vi "programmaticbuild2.vi"() -> ()   [LabVIEW 2015]
doc: "This VI reads an unlimited number of parameters corresponding to project files to build. To build projects programmatically, enter the following text in the command line window to run this VI:\n\n<LabVIEW directory>\\labview.exe \"<this VI>\" -- \"<project file 1>.lvproj\" \"<project file 2>.lvproj\" ... \"<project file n>.lvproj\"\n\nRefer to the block diagram for more information about how this VI executes."
panel:
  out "Built Successfully?":bool
  out "Currently building project":string
  # "Select Help»Show Context Help and move the cursor over the VI icon to display help for this VI."
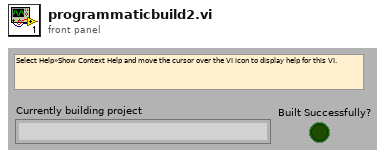
[diagram p1: front panel]
types:
  T1 = enum16{"open", "replace", "create", "open or create", "replace or create", "replace or create with confirmation"}
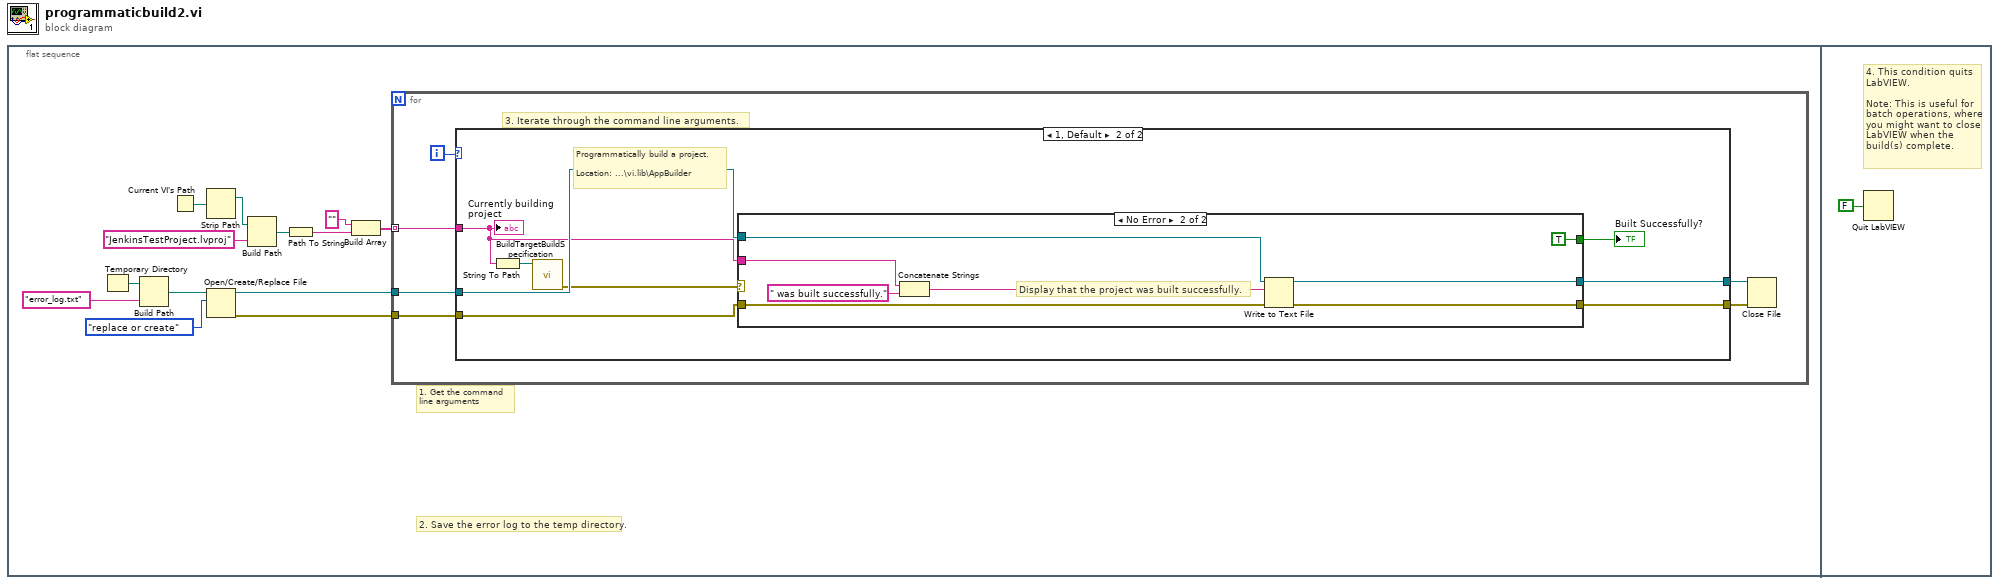
[diagram p0: block diagram]
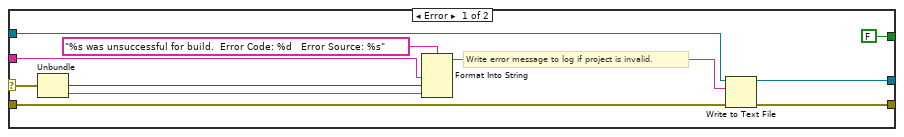
[diagram p3: hidden frame]
diagram:
  n1 = flat-sequence {
    frame #0 {
      # "2. Save the error log to the temp directory."
      # "1. Get the command \nline arguments"
      n2 = Temporary Directory() -> (w10:path)
      n3 = Build Path(base path=w10, name or relative path="error_log.txt") -> (appended path=w8:path)
      n4 = Current VI's Path() -> (path=w5:path)
      n5 = Strip Path(path=w5) -> (stripped path=w4:path)  [unwired: 1 out]
      n6 = Open/Create/Replace File(file path (use dialog)=w8, operation (0:open)=T1."replace or create") -> (refnum out=w12:refnum<file>, error out=w11:errorcluster)  [unwired: 4 in, 1 out]
      n7 = Build Path(base path=w4, name or relative path="JenkinsTestProject.lvproj") -> (appended path=w2:path)
      n8 = Path To String(path=w2) -> (string=w1:string)
      n9 = Build Array("" ("element"), w1) -> (w7:string[])
      n10 = for {
        tunnel: w7 -> [w19] mode=indexing
        tunnel: w12 -> [w17]
        tunnel: w11 -> [w16]
        i -> [w18]
        # "3. Iterate through the command line arguments."
        n11 = case shown="1, Default" w18 {
          tunnel: w19 -> [_ w22]
          tunnel: w17 -> [w21 w28]
          tunnel: w16 -> [w20 w27]
          tunnel: [w20 w26] -> w15
          tunnel: [w21 w25] -> w14
          frame 0 {
            # "The first argument is LabVIEW and is ignored."
          }
          frame 1, Default {
            # "Programmatically build a project.\n\nLocation: ...\\vi.lib\\AppBuilder"
            n12 = String To Path(string=w22) -> (path=w29:path)
            n13 = call <vilib>:"BuildTargetBuildSpecification.vi"("Path to project"=w29) -> ("error out"=w24:errorcluster)  [unwired: 9 in, 1 out]
            n14 = case shown="No Error" w24 {
              selector: w24 -> [w33 _]
              tunnel: w22 -> [w35 w47]
              tunnel: w28 -> [w37 w45]
              tunnel: w27 -> [w40 w44]
              tunnel: [w39 w43] -> w26
              tunnel: [w38 w42] -> w25
              tunnel: [FALSE ("Built Successfully") TRUE ("Built Successfully")] -> w23
              frame Error {
                # "Write error message to log if project is invalid."
                n15 = Unbundle(w33) -> ("code"=w32:i32, "source"=w31:string)  [unwired: 1 out]
                n16 = Format Into String(format string="%s was unsuccessful for build.  Error Code: %d   Error Source: %s" ("string"), w35, w32, w31) -> (resulting string=w34:string)  [unwired: 2 in, 1 out]
                n17 = Write to Text File(file (use dialog)=w37, text=w34, error in=w40) -> (refnum out=w38:refnum<file>, error out=w39:errorcluster)  [unwired: 1 in, 1 out]
              }
              frame No Error {
                # "Display that the project was built successfully."
                n18 = Concatenate Strings "Concatenate Strings"(w47, " was built successfully." ("string")) -> (w46:string)
                n19 = Write to Text File(file (use dialog)=w45, text=w46, error in=w44) -> (refnum out=w42:refnum<file>, error out=w43:errorcluster)  [unwired: 1 in, 1 out]
              }
            }
            "Built Successfully?" <- w23
            "Currently building project" <- w22
          }
        }
        n20 = Close File(refnum=w14, error in=w15) -> ()  [unwired: 2 out]
      }
    }
    frame #1 {
      # "4. This condition quits \nLabVIEW. \n\nNote: This is useful for batch operations, where you might want to close LabVIEW when the build(s) complete."
      n21 = Quit LabVIEW(quit? (T)=FALSE) -> ()
    }
  }
